vi "Periodic Tasks.vi"(11 "error out":errorcluster) -> ()   [LabVIEW 2018]
doc: "This VI runs in parallel to other tasks. It can contain as many user-defined periodic loops as you need. These can carry out PID or other sorts of timed response."
uses:
  <vilib>/Rock Robotics/WPI/Solenoid/WPI_SolenoidValue.ctl
  <vilib>/Rock Robotics/WPI/ThirdParty/Phoenix-LabVIEW/Motor Controller/Controls/CTRE_Phoenix_MotorControl_ControlMode.ctl
  <vilib>/Rock Robotics/WPI/DriverStation/WPI_DriverStationRobotMode2.ctl
  ce0f1a0a-93d2-4219-9beb-48174eeb81d0.vi
  b8a43d1e-5504-4f2a-b76b-f504044aa492.vi
  123062f9-fef7-42b3-b38d-69a70d7ffb4e.vi
  5d4f18ae-01bd-4453-97f8-fc0264503ca9.vi
  df457c05-7057-4a8c-8edf-d82f63e80fbd.vi
  b2a43137-94df-4868-abd1-d49184af5aa7.vi
  e9d14f11-5dad-4d57-98c8-a6c57f493cc1.vi
  035587b2-3d94-40d0-9d42-68c9fbd5af54.vi
  7651e83a-5a2f-4a6d-bbb2-30bf10594118.vi
  RefNums_Actuators.vi
  Motor Power.vi
  RefNumsDriverStation.vi
  Joystick RefNum.vi
  <vilib>/Rock Robotics/WPI/Utilities/WPI_GetSetVariantRefNum.vi
  Robot Global Data.vi
  Robot States.vi
  <vilib>/Rock Robotics/WPI/Solenoid/WPI_SolenoidSetEnum.vi
panel:
  out "Sensor_Loops (ms)":u32
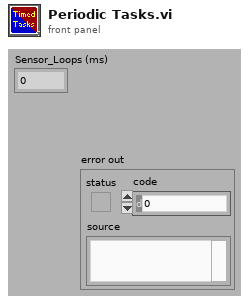
[diagram p1: front panel]
types:
  T1 = typedef "WPI_MotorControlDeviceRef.ctl" = cluster{"DeviceStatus":errorcluster, "Type":T2, "PWM":cluster{"PWM Channel":T3, "DeadBand":T4}, "CAN":cluster{"Device Number":u8, "SetOutput VI Ref":variant, "GetOutput VI Ref":variant, "Enable VI Ref":variant, "Disable VI Ref":variant, "Data":variant}, "Invert":bool, "DIO PWM":cluster{"PWM \"Enable\" Channel":T3, "DIOChannel":T5, "PWM Rate":dbl}}
  T2 = typedef "WPI_MotorControlType.ctl" = enum16{"PWM", "CAN", "DIO PWM"}
  T3 = typedef "FPGA_DIOPWMChannel.ctl" = enum8{"PWM 0", "PWM 1", "PWM 2", "PWM 3", "PWM 4", "PWM 5", "PWM 6", "PWM 7", "PWM 8", "PWM 9", "PWM MXP 0", "PWM MXP 1", "PWM MXP 2", "PWM MXP 3", "PWM MXP 4", "PWM MXP 5", "PWM MXP 6", "PWM MXP 7", "PWM MXP 8", "PWM MXP 9", "Invalid"}
  T4 = typedef "WPI_PWMDeadband.ctl" = cluster{"Name":string, "maxPositivePwm":i32, "minPositivePwm":i32, "centerPwm":i32, "maxNegativePwm":i32, "minNegativePwm":i32, "angularRange":u16}
  T5 = typedef "FPGA_DIOChannel.ctl" = enum8{"DIO 0", "DIO 1", "DIO 2", "DIO 3", "DIO 4", "DIO 5", "DIO 6", "DIO 7", "DIO 8", "DIO 9", "DIO MXP 0", "DIO MXP 1", "DIO MXP 2", "DIO MXP 3", "DIO MXP 4", "DIO MXP 5", "DIO MXP 6", "DIO MXP 7", "DIO MXP 8", "DIO MXP 9", "DIO MXP 10", "DIO MXP 11", "DIO MXP 12", "DIO MXP 13", "DIO MXP 14", "DIO MXP 15", "SPI Port CS1", "SPI Port CS2", "SPI Port CS3", "SPI Port MISO", "SPI Port MOSI", "Invalid"}
  T6 = typedef "WPI_SolenoidDevRef.ctl" = cluster{"DevStatus":errorcluster, "Pneumatics Control Module":u8, "Forward Solenoid Channel":T7, "Reverse Solenoid Channel":T7}
  T7 = typedef "WPI_SolenoidChannel.ctl" = enum8{"Solenoid 0", "Solenoid 1", "Solenoid 2", "Solenoid 3", "Solenoid 4", "Solenoid 5", "Solenoid 6", "Solenoid 7", "Invalid"}
  T8 = typedef "WPI_JoystickDevRef.ctl" = cluster{"Device":T9}
  T9 = typedef "WPI_JoystickDeviceEnum.ctl" = enum16{"USB 0", "USB 1", "USB 2", "USB 3", "USB 4", "USB 5"}
  T10 = typedef "WPI_DriverStationRobotMode2.ctl" = enum16{"Autonomous Disabled", "Autonomous Enabled", "Teleop Disabled", "Teleop Enabled", "Disconnected", "Finish", "Test Disabled", "Test Enabled", "Emergency Stopped"}
  T11 = typedef "CTRE_Phoenix_MotorControl_ControlMode.ctl" = u16
  T12 = typedef "WPI_SolenoidValue.ctl" = enum16{"Off", "On", "Forward", "Reverse"}
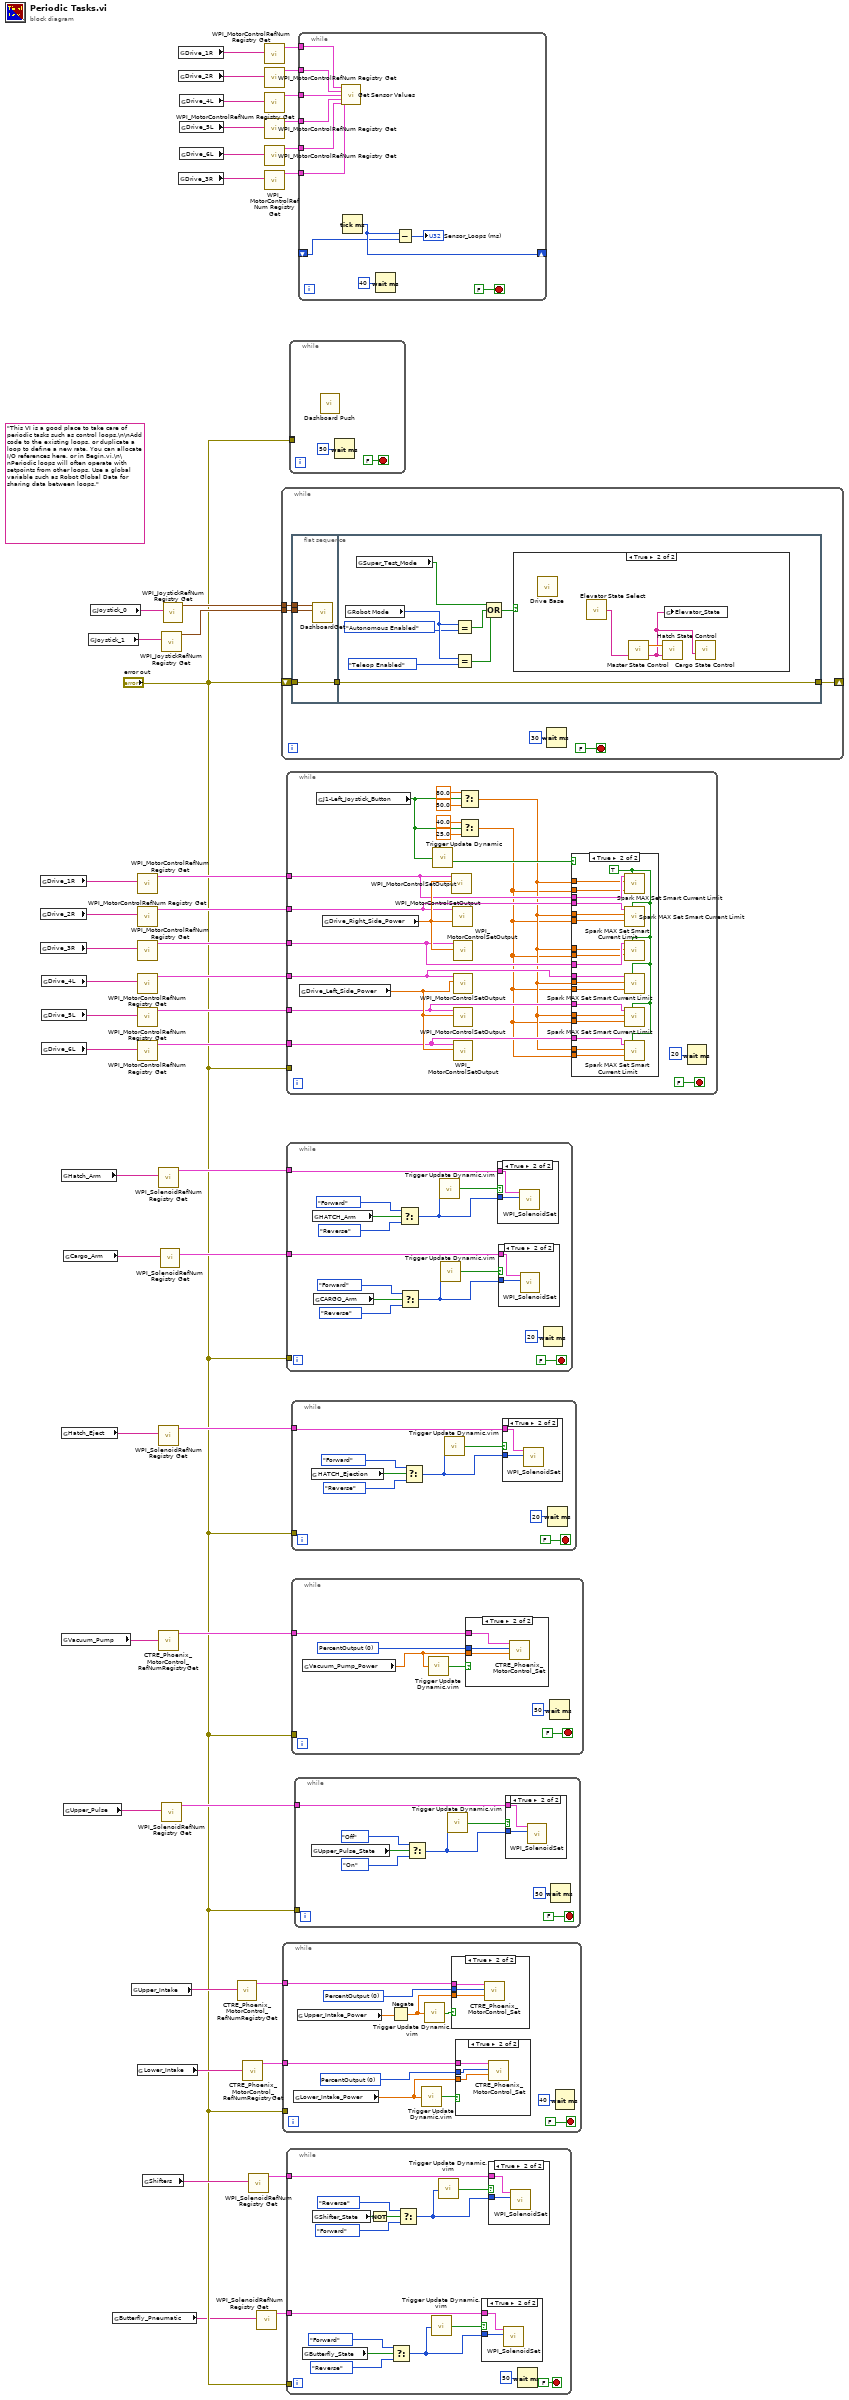
[diagram p0: block diagram]
diagram:
  (unwired) "This VI is a good place to take care of periodic tasks such as control loops.\n\nAdd code to the existing loops, or duplicate a loop to define a new rate. You can allocate I/O references here, or in Begin.vi.\n\nPeriodic loops will often operate with setpoints from other loops. Use a global variable such as Robot Global Data for sharing data between loops."
  n1 = global read "RefNums_Actuators.vi" "Drive_1R"() -> (w47:string)
  n2 = global read "RefNums_Actuators.vi" "Drive_2R"() -> (w46:string)
  n3 = global read "RefNums_Actuators.vi" "Drive_3R"() -> (w45:string)
  n4 = global read "RefNums_Actuators.vi" "Drive_4L"() -> (w44:string)
  n5 = global read "RefNums_Actuators.vi" "Drive_5L"() -> (w43:string)
  n6 = global read "RefNums_Actuators.vi" "Drive_6L"() -> (w42:string)
  n7 = global read "RefNums_Actuators.vi" "Hatch_Arm"() -> (w31:string)
  n8 = global read "RefNums_Actuators.vi" "Hatch_Eject"() -> (w29:string)
  n9 = global read "RefNums_Actuators.vi" "Vacuum_Pump"() -> (w27:string)
  n10 = global read "RefNums_Actuators.vi" "Cargo_Arm"() -> (w23:string)
  n11 = global read "RefNums_Actuators.vi" "Upper_Pulse"() -> (w25:string)
  n12 = global read "Joystick RefNum.vi" "Joystick_1"() -> (w33:string)
  n13 = global read "Joystick RefNum.vi" "Joystick_0"() -> (w35:string)
  n14 = global read "RefNums_Actuators.vi" "Butterfly_Pneumatic"() -> (w2:string)
  n15 = global read "RefNums_Actuators.vi" "Upper_Intake"() -> (w21:string)
  n16 = global read "RefNums_Actuators.vi" "Lower_Intake"() -> (w20:string)
  n17 = call <vilib>:"WPI_MotorControlRefNum Registry Get.vi"("refnum name"=w47) -> ("MotorControlDevRef"=w41:T1)  [unwired: 9 in, 1 out]
  n18 = call <vilib>:"WPI_MotorControlRefNum Registry Get.vi"("refnum name"=w46) -> ("MotorControlDevRef"=w40:T1)  [unwired: 9 in, 1 out]
  n19 = call <vilib>:"WPI_MotorControlRefNum Registry Get.vi"("refnum name"=w45) -> ("MotorControlDevRef"=w39:T1)  [unwired: 9 in, 1 out]
  n20 = call <vilib>:"WPI_MotorControlRefNum Registry Get.vi"("refnum name"=w44) -> ("MotorControlDevRef"=w38:T1)  [unwired: 9 in, 1 out]
  n21 = call <vilib>:"WPI_MotorControlRefNum Registry Get.vi"("refnum name"=w43) -> ("MotorControlDevRef"=w37:T1)  [unwired: 9 in, 1 out]
  n22 = call <vilib>:"WPI_MotorControlRefNum Registry Get.vi"("refnum name"=w42) -> ("MotorControlDevRef"=w36:T1)  [unwired: 9 in, 1 out]
  n23 = global read "RefNums_Actuators.vi" "Shifters"() -> (w5:string)
  n24 = call <vilib>:"WPI_SolenoidRefNum Registry Get.vi"("refnum name"=w31) -> ("SolenoidDevRef"=w30:T6)  [unwired: 9 in, 1 out]
  n25 = call <vilib>:"WPI_SolenoidRefNum Registry Get.vi"("refnum name"=w29) -> ("SolenoidDevRef"=w28:T6)  [unwired: 9 in, 1 out]
  n26 = call <vilib>:"CTRE_Phoenix_MotorControl_RefNumRegistryGet.vi"("refnum name"=w27) -> ("PhoenixMotorControlDevRef"=w26:T1)  [unwired: 9 in, 1 out]
  n27 = call <vilib>:"WPI_SolenoidRefNum Registry Get.vi"("refnum name"=w23) -> ("SolenoidDevRef"=w22:T6)  [unwired: 9 in, 1 out]
  n28 = call <vilib>:"WPI_JoystickRefNum Registry Get.vi"("refnum name"=w33) -> ("JoystickDevRef"=w32:T8)  [unwired: 9 in, 1 out]
  n29 = call <vilib>:"WPI_SolenoidRefNum Registry Get.vi"("refnum name"=w25) -> ("SolenoidDevRef"=w24:T6)  [unwired: 9 in, 1 out]
  n30 = call <vilib>:"WPI_JoystickRefNum Registry Get.vi"("refnum name"=w35) -> ("JoystickDevRef"=w34:T8)  [unwired: 9 in, 1 out]
  n31 = global read "RefNums_Actuators.vi" "Drive_1R"() -> (w17:string)
  n32 = global read "RefNums_Actuators.vi" "Drive_2R"() -> (w16:string)
  n33 = global read "RefNums_Actuators.vi" "Drive_3R"() -> (w12:string)
  n34 = global read "RefNums_Actuators.vi" "Drive_4L"() -> (w15:string)
  n35 = global read "RefNums_Actuators.vi" "Drive_5L"() -> (w14:string)
  n36 = global read "RefNums_Actuators.vi" "Drive_6L"() -> (w13:string)
  n37 = call <vilib>:"CTRE_Phoenix_MotorControl_RefNumRegistryGet.vi"("refnum name"=w21) -> ("PhoenixMotorControlDevRef"=w19:T1)  [unwired: 9 in, 1 out]
  n38 = call <vilib>:"CTRE_Phoenix_MotorControl_RefNumRegistryGet.vi"("refnum name"=w20) -> ("PhoenixMotorControlDevRef"=w18:T1)  [unwired: 9 in, 1 out]
  n39 = call <vilib>:"WPI_SolenoidRefNum Registry Get.vi"("refnum name"=w5) -> ("SolenoidDevRef"=w4:T6)  [unwired: 9 in, 1 out]
  n40 = call <vilib>:"WPI_SolenoidRefNum Registry Get.vi"("refnum name"=w2) -> ("SolenoidDevRef"=w1:T6)  [unwired: 9 in, 1 out]
  n41 = call <vilib>:"WPI_MotorControlRefNum Registry Get.vi"("refnum name"=w17) -> ("MotorControlDevRef"=w11:T1)  [unwired: 9 in, 1 out]
  n42 = call <vilib>:"WPI_MotorControlRefNum Registry Get.vi"("refnum name"=w16) -> ("MotorControlDevRef"=w10:T1)  [unwired: 9 in, 1 out]
  n43 = call <vilib>:"WPI_MotorControlRefNum Registry Get.vi"("refnum name"=w15) -> ("MotorControlDevRef"=w9:T1)  [unwired: 9 in, 1 out]
  n44 = call <vilib>:"WPI_MotorControlRefNum Registry Get.vi"("refnum name"=w14) -> ("MotorControlDevRef"=w8:T1)  [unwired: 9 in, 1 out]
  n45 = call <vilib>:"WPI_MotorControlRefNum Registry Get.vi"("refnum name"=w13) -> ("MotorControlDevRef"=w7:T1)  [unwired: 9 in, 1 out]
  n46 = call <vilib>:"WPI_MotorControlRefNum Registry Get.vi"("refnum name"=w12) -> ("MotorControlDevRef"=w6:T1)  [unwired: 9 in, 1 out]
  n47 = while {
    tunnel: w34 -> [w52]
    tunnel: w32 -> [w51]
    shift-right: [w50] -> _
    shift-left: "error out" -> [w48]
    stop <- FALSE stop-if-true
    n48 = flat-sequence {
      tunnel: w52 -> [w57]
      tunnel: w51 -> [w56]
      tunnel: [w55] -> w49
      tunnel: w48 -> [w55]
      tunnel: [w58] -> w50
      tunnel: w49 -> [w58]
      frame #0 {
        n49 = call "DashboardGet.vi"("Joystick 2"=w56, "Joystick 1"=w57) -> ()  [unwired: 10 in]
      }
      frame #1 {
        n50 = global read "Robot Global Data.vi" "Robot Mode"() -> (w64:T10)
        n51 = global read "RefNumsDriverStation.vi" "Super_Test_Mode"() -> (w65:bool)
        n52 = Equal?(x=w64, y=WPI_DriverStationRobotMode2."Autonomous Enabled") -> (x = y?=w61:bool)
        n53 = Equal?(x=w64, y=WPI_DriverStationRobotMode2."Teleop Enabled") -> (x = y?=w60:bool)
        n54 = Compound Arithmetic op=OR(w65, w61, w60) -> (w59:bool)
        n55 = case shown="True" w59 {
          frame False {
          }
          frame True {
            n56 = call "Drive Base.vi"() -> ()  [unwired: 12 in]
            n57 = call "Elevator State Select.vi"() -> ("Elevator_State"=w68:string)  [unwired: 2 in]
            n58 = call "Master State Control.vi"("Elevator_State"=w68) -> ("Elevator_State_Out"=w66:string, "Target_Vacuum_Pump_Power"=w67:dbl)  [unwired: 1 in]
            n59 = call "Hatch State Control.vi"("Elevator State"=w66, "Vacuum Pump Power"=w67) -> ()  [unwired: 2 in]
            n60 = global write "Robot States.vi" "Elevator_State"(w66) -> ()
            n61 = call "Cargo State Control.vi"("Elevator State"=w66) -> ()  [unwired: 11 in]
          }
        }
      }
    }
    n62 = Wait (ms)(milliseconds to wait=u32 30) -> ()  [unwired: 1 out]
  }
  n63 = while {
    tunnel: w19 -> [w77]
    tunnel: w18 -> [w71]
    tunnel: "error out" -> [_]
    stop <- FALSE stop-if-true
    w70 = T11 0 items=["PercentOutput"=0, "Position"=1, "Velocity"=2, "Current"=3, "Follower"=5, "MotionProfile"=6, "MotionMagic"=7, "MotionProfileArc"=10, "Disabled"=15] ("Control Mode")
    w76 = T11 0 items=["PercentOutput"=0, "Position"=1, "Velocity"=2, "Current"=3, "Follower"=5, "MotionProfile"=6, "MotionMagic"=7, "MotionProfileArc"=10, "Disabled"=15] ("Control Mode")
    n64 = global read "Motor Power.vi" "Lower_Intake_Power"() -> (w69:dbl)
    n65 = global read "Motor Power.vi" "Upper_Intake_Power"() -> (w75:dbl)
    n66 = Negate(x=w75) -> (-x=w74:dbl)
    n67 = call "Trigger Update Dynamic.vim"("Trigger"=w69) -> ("Update"=w72:bool)
    n68 = call "Trigger Update Dynamic.vim"("Trigger"=w74) -> ("Update"=w73:bool)
    n69 = case shown="True" w73 {
      tunnel: w77 -> [_ w85]
      tunnel: w76 -> [_ w84]
      tunnel: w74 -> [_ w83]
      frame False {
      }
      frame True {
        n70 = call <vilib>:"CTRE_Phoenix_MotorControl_Set.vi"("Output"=w83, "Control Mode"=w84, "PhoenixMotorControlDevRef"=w85) -> ()  [unwired: 7 in, 2 out]
      }
    }
    n71 = case shown="True" w72 {
      tunnel: w71 -> [_ w82]
      tunnel: w70 -> [_ w81]
      tunnel: w69 -> [_ w80]
      frame False {
      }
      frame True {
        n72 = call <vilib>:"CTRE_Phoenix_MotorControl_Set.vi"("Output"=w80, "Control Mode"=w81, "PhoenixMotorControlDevRef"=w82) -> ()  [unwired: 7 in, 2 out]
      }
    }
    n73 = Wait (ms)(milliseconds to wait=u32 40) -> ()  [unwired: 1 out]
  }
  n74 = while {
    tunnel: w41 -> [w93]
    tunnel: w40 -> [w92]
    tunnel: w39 -> [w91]
    tunnel: w38 -> [w90]
    tunnel: w37 -> [w89]
    tunnel: w36 -> [w88]
    tunnel: "error out" -> [_]
    stop <- FALSE stop-if-true
    n75 = global read "Motor Power.vi" "Drive_Left_Side_Power"() -> (w102:dbl)
    n76 = global read "RefNumsDriverStation.vi" "J1-Left_Joystick_Button"() -> (w95:bool)
    n77 = global read "Motor Power.vi" "Drive_Right_Side_Power"() -> (w103:dbl)
    n78 = call "Trigger Update Dynamic.vi"("Trigger"=w95) -> ("Update"=w94:bool)
    n79 = call <vilib>:"WPI_MotorControlSetOutput.vi"("Output"=w103, "MotorControlDevRef"=w93) -> ()  [unwired: 7 in, 3 out]
    n80 = call <vilib>:"WPI_MotorControlSetOutput.vi"("Output"=w103, "MotorControlDevRef"=w92) -> ()  [unwired: 7 in, 3 out]
    n81 = call <vilib>:"WPI_MotorControlSetOutput.vi"("Output"=w103, "MotorControlDevRef"=w91) -> ()  [unwired: 7 in, 3 out]
    n82 = call <vilib>:"WPI_MotorControlSetOutput.vi"("Output"=w102, "MotorControlDevRef"=w90) -> ()  [unwired: 7 in, 3 out]
    n83 = call <vilib>:"WPI_MotorControlSetOutput.vi"("Output"=w102, "MotorControlDevRef"=w89) -> ()  [unwired: 7 in, 3 out]
    n84 = call <vilib>:"WPI_MotorControlSetOutput.vi"("Output"=w102, "MotorControlDevRef"=w88) -> ()  [unwired: 7 in, 3 out]
    n85 = Select(t=80.0, s=w95, f=50.0) -> (s? t:f=w87:dbl)
    n86 = Select(t=40.0, s=w95, f=25.0) -> (s? t:f=w86:dbl)
    n87 = case shown="True" w94 {
      tunnel: w93 -> [_ w122]
      tunnel: w92 -> [_ w121]
      tunnel: w91 -> [_ w120]
      tunnel: w90 -> [_ w119]
      tunnel: w89 -> [_ w118]
      tunnel: w88 -> [_ w117]
      tunnel: w87 -> [_ w116]
      tunnel: w87 -> [_ w115]
      tunnel: w87 -> [_ w114]
      tunnel: w87 -> [_ w113]
      tunnel: w87 -> [_ w112]
      tunnel: w87 -> [_ w111]
      tunnel: w86 -> [_ w110]
      tunnel: w86 -> [_ w109]
      tunnel: w86 -> [_ w108]
      tunnel: w86 -> [_ w107]
      tunnel: w86 -> [_ w106]
      tunnel: w86 -> [_ w105]
      frame False {
      }
      frame True {
        w104 = TRUE ("Linearized Limit Enabled (F)")
        n88 = call <vilib>:"Spark MAX Set Smart Current Limit.vi"("Linearized Limit Enabled (F)"=w104, "Free Speed Current Limit (20A)"=w110, "Primay Current Limit (80A)"=w116, "MotorControlDeviceRef in"=w122) -> ()  [unwired: 6 in, 2 out]
        n89 = call <vilib>:"Spark MAX Set Smart Current Limit.vi"("Linearized Limit Enabled (F)"=w104, "Free Speed Current Limit (20A)"=w109, "Primay Current Limit (80A)"=w115, "MotorControlDeviceRef in"=w121) -> ()  [unwired: 6 in, 2 out]
        n90 = call <vilib>:"Spark MAX Set Smart Current Limit.vi"("Linearized Limit Enabled (F)"=w104, "Free Speed Current Limit (20A)"=w108, "Primay Current Limit (80A)"=w114, "MotorControlDeviceRef in"=w120) -> ()  [unwired: 6 in, 2 out]
        n91 = call <vilib>:"Spark MAX Set Smart Current Limit.vi"("Linearized Limit Enabled (F)"=w104, "Free Speed Current Limit (20A)"=w107, "Primay Current Limit (80A)"=w113, "MotorControlDeviceRef in"=w119) -> ()  [unwired: 6 in, 2 out]
        n92 = call <vilib>:"Spark MAX Set Smart Current Limit.vi"("Linearized Limit Enabled (F)"=w104, "Free Speed Current Limit (20A)"=w106, "Primay Current Limit (80A)"=w112, "MotorControlDeviceRef in"=w118) -> ()  [unwired: 6 in, 2 out]
        n93 = call <vilib>:"Spark MAX Set Smart Current Limit.vi"("Linearized Limit Enabled (F)"=w104, "Free Speed Current Limit (20A)"=w105, "Primay Current Limit (80A)"=w111, "MotorControlDeviceRef in"=w117) -> ()  [unwired: 6 in, 2 out]
      }
    }
    n94 = Wait (ms)(milliseconds to wait=u32 20) -> ()  [unwired: 1 out]
  }
  n95 = while {
    tunnel: w30 -> [w135]
    tunnel: "error out" -> [_]
    tunnel: w22 -> [w123]
    stop <- FALSE stop-if-true
    n96 = global read "Robot States.vi" "HATCH_Arm"() -> (w136:bool)
    n97 = global read "Robot States.vi" "CARGO_Arm"() -> (w128:bool)
    n98 = Select(t=WPI_SolenoidValue."Forward" ("Value"), s=w136, f=WPI_SolenoidValue."Reverse" ("Value")) -> (s? t:f=w131:T12)
    n99 = Select(t=WPI_SolenoidValue."Forward" ("Value"), s=w128, f=WPI_SolenoidValue."Reverse" ("Value")) -> (s? t:f=w126:T12)
    n100 = call "Trigger Update Dynamic.vim"("Trigger"=w131) -> ("Update"=w134:bool)
    n101 = call "Trigger Update Dynamic.vim"("Trigger"=w126) -> ("Update"=w127:bool)
    n102 = case shown="True" w134 {
      tunnel: w135 -> [_ w140]
      tunnel: w131 -> [_ w139]
      frame False {
      }
      frame True {
        n103 = call-poly <vilib>:"WPI_SolenoidSet.vi"("Value"=w139, "SolenoidDevRef"=w140) -> ()  [unwired: 8 in, 2 out]
      }
    }
    n104 = case shown="True" w127 {
      tunnel: w123 -> [_ w138]
      tunnel: w126 -> [_ w137]
      frame False {
      }
      frame True {
        n105 = call-poly <vilib>:"WPI_SolenoidSet.vi"("Value"=w137, "SolenoidDevRef"=w138) -> ()  [unwired: 8 in, 2 out]
      }
    }
    n106 = Wait (ms)(milliseconds to wait=u32 20) -> ()  [unwired: 1 out]
  }
  n107 = while {
    tunnel: w4 -> [w147]
    tunnel: "error out" -> [_]
    tunnel: w1 -> [w142]
    stop <- FALSE stop-if-true
    n108 = global read "Robot States.vi" "Butterfly_State"() -> (w141:bool)
    n109 = global read "Robot States.vi" "Shifter_State"() -> (w155:bool)
    n110 = Not(x=w155) -> (.not. x?=w150:bool)
    n111 = Select(t=WPI_SolenoidValue."Forward" ("Value"), s=w141, f=WPI_SolenoidValue."Reverse" ("Value")) -> (s? t:f=w145:T12)
    n112 = Select(t=WPI_SolenoidValue."Reverse" ("Value"), s=w150, f=WPI_SolenoidValue."Forward" ("Value")) -> (s? t:f=w153:T12)
    n113 = call "Trigger Update Dynamic.vim"("Trigger"=w145) -> ("Update"=w146:bool)
    n114 = call "Trigger Update Dynamic.vim"("Trigger"=w153) -> ("Update"=w154:bool)
    n115 = case shown="True" w146 {
      tunnel: w145 -> [_ w157]
      tunnel: w142 -> [_ w156]
      frame False {
      }
      frame True {
        n116 = call-poly <vilib>:"WPI_SolenoidSet.vi"("Value"=w157, "SolenoidDevRef"=w156) -> ()  [unwired: 8 in, 2 out]
      }
    }
    n117 = case shown="True" w154 {
      tunnel: w153 -> [_ w159]
      tunnel: w147 -> [_ w158]
      frame False {
      }
      frame True {
        n118 = call-poly <vilib>:"WPI_SolenoidSet.vi"("Value"=w159, "SolenoidDevRef"=w158) -> ()  [unwired: 8 in, 2 out]
      }
    }
    n119 = Wait (ms)(milliseconds to wait=u32 50) -> ()  [unwired: 1 out]
  }
  n120 = while {
    tunnel: [w160] -> _
    tunnel: "error out" -> [w160]
    stop <- FALSE stop-if-true
    n121 = call "Dashboard Push.vi"() -> ()  [unwired: 12 in]
    n122 = Wait (ms)(milliseconds to wait=u32 50) -> ()  [unwired: 1 out]
  }
  n123 = while {
    tunnel: w28 -> [w169]
    tunnel: "error out" -> [_]
    stop <- FALSE stop-if-true
    n124 = global read "Robot States.vi" "HATCH_Ejection"() -> (w170:bool)
    n125 = Select(t=WPI_SolenoidValue."Forward" ("Value"), s=w170, f=WPI_SolenoidValue."Reverse" ("Value")) -> (s? t:f=w165:T12)
    n126 = call "Trigger Update Dynamic.vim"("Trigger"=w165) -> ("Update"=w168:bool)
    n127 = case shown="True" w168 {
      tunnel: w169 -> [_ w172]
      tunnel: w165 -> [_ w171]
      frame False {
      }
      frame True {
        n128 = call-poly <vilib>:"WPI_SolenoidSet.vi"("Value"=w171, "SolenoidDevRef"=w172) -> ()  [unwired: 8 in, 2 out]
      }
    }
    n129 = Wait (ms)(milliseconds to wait=u32 20) -> ()  [unwired: 1 out]
  }
  n130 = while {
    tunnel: w26 -> [w175]
    tunnel: "error out" -> [_]
    stop <- FALSE stop-if-true
    w176 = T11 0 items=["PercentOutput"=0, "Position"=1, "Velocity"=2, "Current"=3, "Follower"=5, "MotionProfile"=6, "MotionMagic"=7, "MotionProfileArc"=10, "Disabled"=15] ("Control Mode")
    n131 = global read "Robot States.vi" "Vacuum_Pump_Power"() -> (w177:dbl)
    n132 = call "Trigger Update Dynamic.vim"("Trigger"=w177) -> ("Update"=w178:bool)
    n133 = case shown="True" w178 {
      tunnel: w177 -> [_ w181]
      tunnel: w176 -> [_ w180]
      tunnel: w175 -> [_ w179]
      frame False {
      }
      frame True {
        n134 = call <vilib>:"CTRE_Phoenix_MotorControl_Set.vi"("Output"=w181, "Control Mode"=w180, "PhoenixMotorControlDevRef"=w179) -> ()  [unwired: 7 in, 2 out]
      }
    }
    n135 = Wait (ms)(milliseconds to wait=u32 50) -> ()  [unwired: 1 out]
  }
  n136 = while {
    tunnel: w24 -> [w188]
    tunnel: "error out" -> [_]
    stop <- FALSE stop-if-true
    n137 = global read "Robot States.vi" "Upper_Pulse_State"() -> (w189:bool)
    n138 = Select(t=WPI_SolenoidValue."Off" ("Value"), s=w189, f=WPI_SolenoidValue."On" ("Value")) -> (s? t:f=w184:T12)
    n139 = call "Trigger Update Dynamic.vim"("Trigger"=w184) -> ("Update"=w187:bool)
    n140 = case shown="True" w187 {
      tunnel: w188 -> [_ w191]
      tunnel: w184 -> [_ w190]
      frame False {
      }
      frame True {
        n141 = call-poly <vilib>:"WPI_SolenoidSet.vi"("Value"=w190, "SolenoidDevRef"=w191) -> ()  [unwired: 8 in, 2 out]
      }
    }
    n142 = Wait (ms)(milliseconds to wait=u32 50) -> ()  [unwired: 1 out]
  }
  n143 = while {
    tunnel: w11 -> [w200]
    tunnel: w10 -> [w199]
    tunnel: w9 -> [w198]
    tunnel: w8 -> [w197]
    tunnel: w7 -> [w196]
    tunnel: w6 -> [w195]
    shift-right: [w194] -> _
    shift-left: _ -> [w193]
    stop <- FALSE stop-if-true
    n144 = call "Get Sensor Values.vi"("Ref_Drive 1R"=w200, "Ref_Drive 2R"=w199, "Ref_Drive 4L"=w198, "Ref_Drive 5L"=w197, "Ref_Drive 6L"=w196, "Ref_Drive 3R"=w195) -> ()  [unwired: 10 in]
    n145 = Tick Count (ms)() -> (millisecond timer value=w194:u32)
    n146 = Wait (ms)(milliseconds to wait=u32 40) -> ()  [unwired: 1 out]
    n147 = Subtract(x=w194, y=w193) -> (x-y=→"Sensor_Loops (ms)":u32)
  }
